vi "IB_Load_Class.vi"(8 "error in (no error)":errorcluster, 11 "IB_Class path":path) -> (0 "error out":errorcluster, 3 "IB_Installer out":refnum<class "Installer.lvclass">)   [LabVIEW 2020]
uses:
  <vilib>/AppBuilder/IB_Classes/Installer/Installer.lvclass
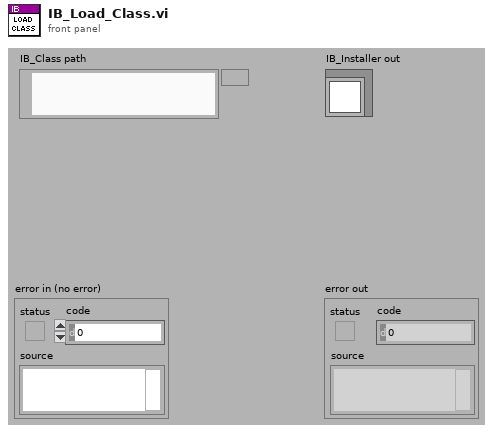
[diagram p1: front panel]
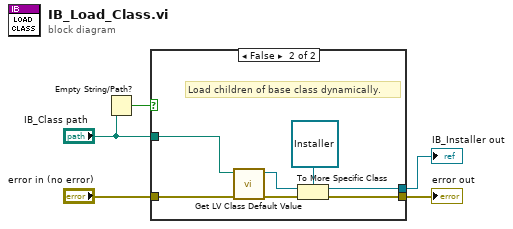
[diagram p0: block diagram]
diagram:
  n1 = Empty String/Path?(string/path="IB_Class path") -> (empty?=w2:bool)
  n2 = case shown="False" w2 {
    tunnel: [_ w13] -> w5
    tunnel: "error in (no error)" -> [w6 w12]
    tunnel: [w6 w11] -> w3
    tunnel: "IB_Class path" -> [_ w8]
    frame True {
      # "Source Distribution"
      # "If path is not valid, return default base class object."
    }
    frame False {
      # "Load children of base class dynamically."
      n3 = call <vilib>:"Get LV Class Default Value.vi"("error in (no error)"=w12, "class path"=w8) -> ("error out"=w10:errorcluster, "object"=w9:refnum<class>)  [unwired: 8 out]
      n4 = To More Specific Class(target class=refnum<class "Installer.lvclass"> refnum ("Installer.lvclass"), reference=w9, error in=w10) -> (specific class reference=w13:refnum<class "Installer.lvclass">, error out=w11:errorcluster)
    }
  }
  "IB_Installer out" <- w5
  "error out" <- w3
